vi "Get Service Descriptor.vi"(8 "error in":errorcluster, 11 "measurement plugin service in":refnum<class "Measurement Plugin Service.lvclass">) -> (0 "error out":errorcluster, 2 "service descriptor":T1, 3 "measurement plugin service out":refnum<class "Measurement Plugin Service.lvclass">)   [LabVIEW 2021, in "NI Measurement Plug-In SDK.lvlib" / "Measurement Plugin Service.lvclass"]
uses:
  Measurement Plugin Service.lvclass
  Helpers/TypeDefs/Service Descriptor.ctl
  Helpers/TypeDefs/Measurement Details.ctl
  Helpers/TypeDefs/Measurement Annotation.ctl
  NI Measurement Plug-In SDK.lvlib
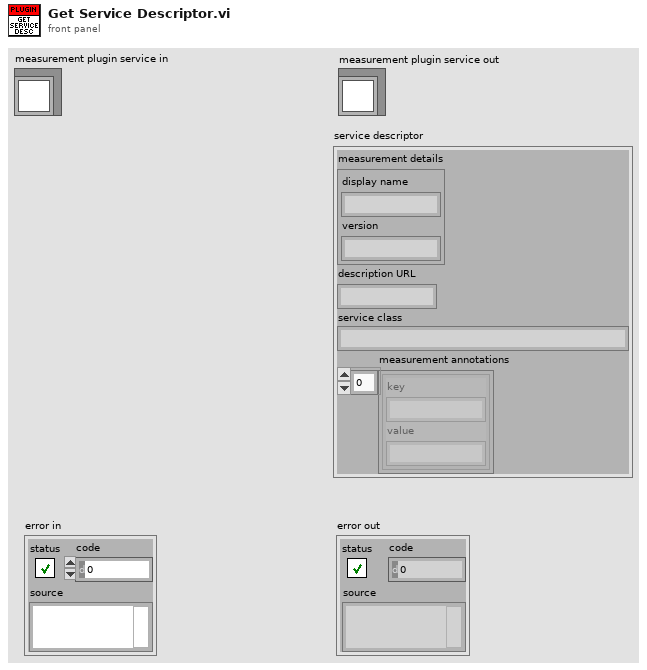
[diagram p1: front panel]
types:
  T1 = typedef "NI Measurement Plug-In SDK.lvlib/Service Descriptor.ctl" = cluster{"measurement details":T2, "description URL":string, "service class":string, "measurement annotations":T3[]}
  T2 = typedef "NI Measurement Plug-In SDK.lvlib/Measurement Details.ctl" = cluster{"display name":string, "version":string}
  T3 = typedef "NI Measurement Plug-In SDK.lvlib/Measurement Annotation.ctl" = cluster{"key":string, "value":string}
  T4 = typedef "NI Measurement Plug-In SDK.lvlib/Measurement Plugin Service.lvclass/Plugin Paths.ctl" = cluster{"get service descriptor VI path":path, "get type specializations VI path":path, "get UI details VI path":path, "measurement logic VI path":path, "measurement configuration ctl path":path, "measurement results ctl path":path}
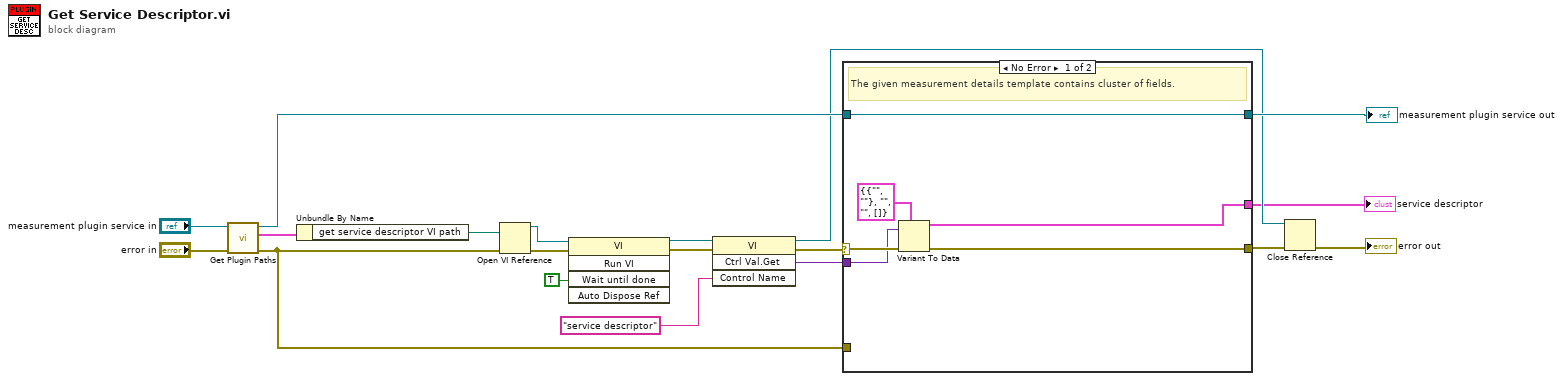
[diagram p0: block diagram]
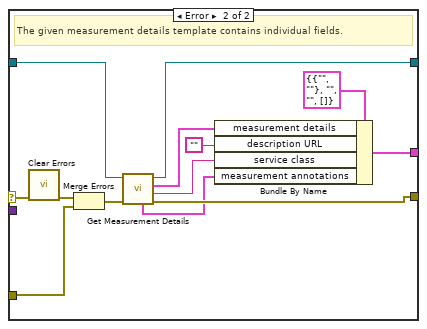
[diagram p2: hidden frame]
diagram:
  n1 = call-dynamic "Get Plugin Paths.vi"("error in"="error in", "measurement plugin service in"="measurement plugin service in") -> ("error out"=w9:errorcluster, "plugin paths"=w19:T4, "measurement plugin service out"=w8:refnum<class "Measurement Plugin Service.lvclass">)  [unwired: 7 in]
  n2 = Unbundle By Name(w19) -> ("get service descriptor VI path"=w18:path)
  n3 = Open VI Reference(vi path=w18, error in (no error)=w9) -> (vi reference=w16:refnum<vi>, error out=w17:errorcluster)  [unwired: 4 in]
  n4 = invoke class="VI" method="Run VI"(reference=w16, error in=w17, "Wait until done"=TRUE ("Wait Until Done")) -> (reference out=w13:refnum<vi>, error out=w14:errorcluster)  [unwired: 2 in, 3 out]
  n5 = invoke class="VI" method="Ctrl Val.Get"(reference=w13, error in=w14, "Control Name"="service descriptor") -> (reference out=w3:refnum<vi>, error out=w11:errorcluster, "Get Control Value Variant"=w10:variant)  [unwired: 1 in, 1 out]
  n6 = case shown="No Error" w11 {
    selector: w11 -> [w25 w38]
    tunnel: w10 -> [w24 _]
    tunnel: w9 -> [_ w36]
    tunnel: [w22 w34] -> w5
    tunnel: [w21 w32] -> w4
    tunnel: w8 -> [w21 w33]
    tunnel: [w20 w27] -> w2
    frame No Error {
      # "The given measurement details template contains cluster of fields."
      n7 = Variant To Data(error in=w25, type=T1 {"measurement details"={"display name"="", "version"=""}, "description URL"="", "service class"="", "measurement annotations"=[]} ("service descriptor"), Variant=w24) -> (data=w20:T1, error out=w22:errorcluster)
    }
    frame Error {
      # "The given measurement details template contains individual fields."
      n8 = call <vilib>:"Clear Errors.vi"("error in (no error)"=w38) -> ("error out"=w37:errorcluster)  [unwired: 5 in, 1 out]
      n9 = Merge Errors(w37, w36) -> (w35:errorcluster)
      n10 = call-dynamic "Get Measurement Details.vi"("error in"=w35, "measurement plugin service in"=w33) -> ("error out"=w34:errorcluster, "service class"=w29:string, "measurement details"=w31:T2, "measurement plugin service out"=w32:refnum<class "Measurement Plugin Service.lvclass">, "measurement annotations"=w28:T3[])  [unwired: 5 in]
      n11 = Bundle By Name(cluster=T1 {"measurement details"={"display name"="", "version"=""}, "description URL"="", "service class"="", "measurement annotations"=[]} ("service descriptor"), "measurement details"=w31, "description URL"="", "service class"=w29, "measurement annotations"=w28) -> (w27:T1)
    }
  }
  "measurement plugin service out" <- w4
  "service descriptor" <- w2
  n12 = Close Reference(reference=w3, error in (no error)=w5) -> (error out=→"error out":errorcluster)
